vi "Shutdown.vi"(4 "error in (no error)":errorcluster, 7 "CmdLib In":refnum<k24>) -> (0 "error out":errorcluster, 3 "CmdLib Out":refnum<k24>)   [LabVIEW 2009]
uses:
  C:/Code/Apps/Utilities/Picomotor/PicomotorApp/Install/Samples/LabVIEW/Model 8742/LabVIEW 2009/CmdLib.dll
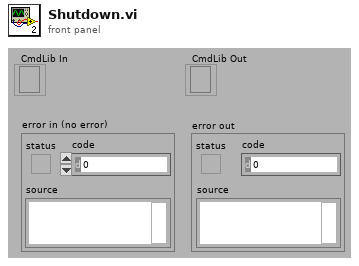
[diagram p1: front panel]
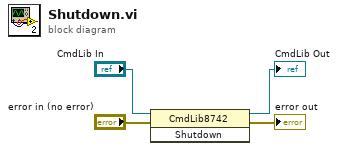
[diagram p0: block diagram]
diagram:
  n1 = invoke class="CmdLib8742" method="Shutdown"(reference="CmdLib In", error in="error in (no error)") -> (reference out=→"CmdLib Out":refnum<k24>, error out=→"error out":errorcluster)  [unwired: 1 in, 1 out]
